vi "determineNewTestLogFilePath.vi"(8 "error in (no error)":errorcluster, 11 "Logger in":refnum<class "Logger.lvclass">) -> (0 "error out":errorcluster, 2 "logFilePath":path, 3 "Logger out":refnum<class "Logger.lvclass">)   [LabVIEW 2013, in "Logger.lvclass"]
uses:
  Logger.lvclass
  Logger.lvclass/Logger.ctl
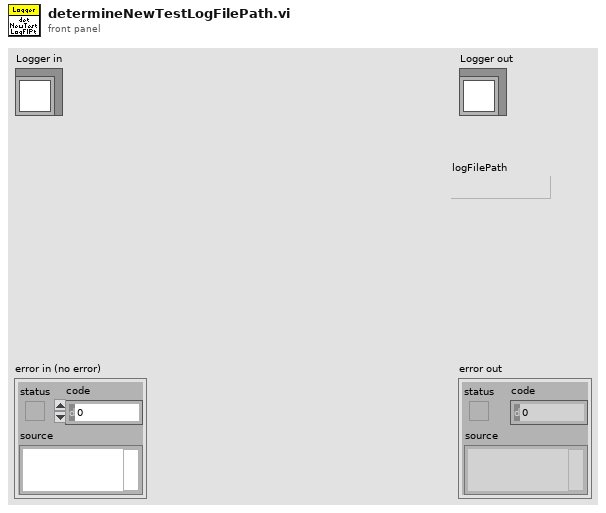
[diagram p1: front panel]
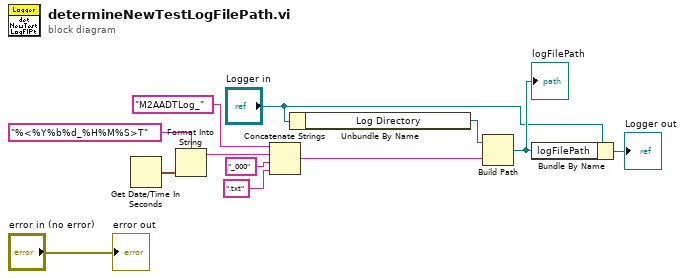
[diagram p0: block diagram]
diagram:
  n1 = Get Date/Time In Seconds() -> (seconds since 1Jan1904=w7:timestamp)
  n2 = Format Into String(format string="%<%Y%b%d_%H%M%S>T", w7) -> (resulting string=w10:string)  [unwired: 2 in, 1 out]
  n3 = Concatenate Strings("M2AADTLog_" ("string"), w10, "_000" ("string"), ".txt" ("string")) -> (w8:string)
  n4 = Unbundle By Name("Logger in") -> ("Log Directory"=w2:path)
  n5 = Build Path(base path=w2, name or relative path=w8) -> (appended path=w4:path)
  "logFilePath" <- w4
  n6 = Bundle By Name(cluster="Logger in", "logFilePath"=w4) -> (→"Logger out":refnum<class "Logger.lvclass">)
  "error out" <- "error in (no error)"
